vi "toString.vi"(10 "Variant":variant, 11 "StringFormatter in":refnum<class "StringFormatter.lvclass">) -> (0 "error out":errorcluster, 2 "Value":string)   [LabVIEW 2013, in "OpenStringFormatter.lvlib" / "StringFormatter.lvclass"]
uses:
  StringFormatter.lvclass
  StringFormatter.lvclass/StringFormatter.ctl
  TypeDescriptor/OpenDescriptor.lvlib
  Conversions/OpenConvert.lvlib
  Variant/OpenVariant.lvlib
panel:
  out "interleaved array (noUnits)":u8[](array[numeric]) format="%.0x"
  out "x = y?":bool
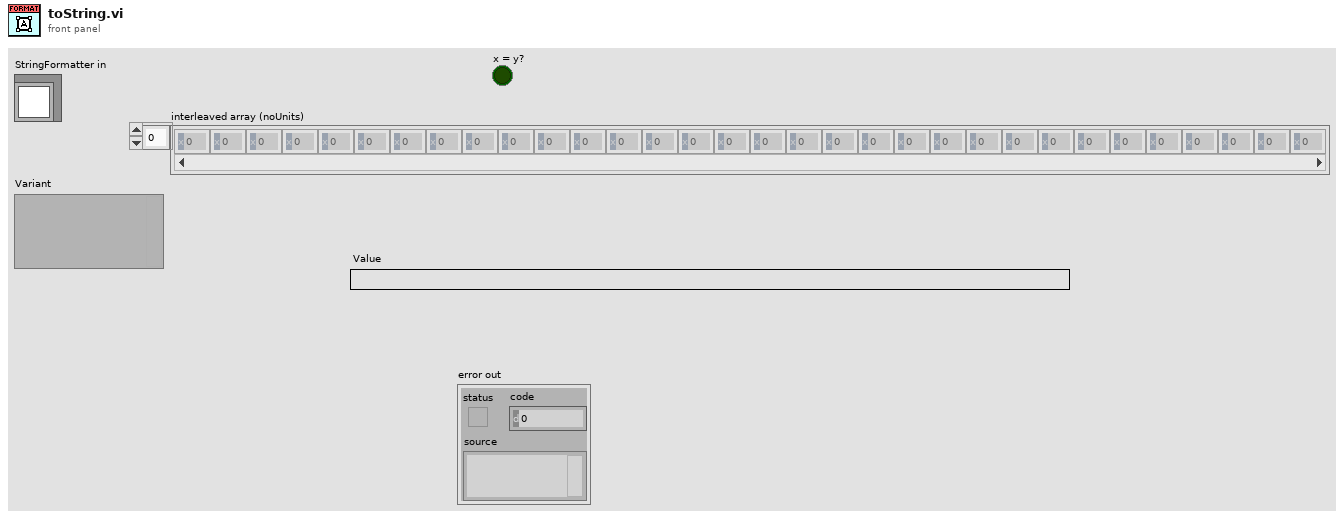
[diagram p1: front panel]
types:
  T1 = typedef "OpenStringFormatter.lvlib/StringFormatter.lvclass/Localization Decimal Separator -- enum.ctl" = enum16{"System", "Comma", "Dot"}
  T2 = typedef "VariantType.lvlib/UnitInfo.ctl" = cluster{"UnitType":T3, "Exponent":i16}
  T3 = typedef "VariantType.lvlib/UnitType.ctl" = enum16{"Radians", "Steradians", "Seconds", "Meters", "Kilograms", "Amperes", "Kelvins", "Moles", "Candelas", "InvalidUnit"}
  T4 = typedef "Type Enum.ctl" = enum8{"Void", "I8", "I16", "I32", "I64", "U8", "U16", "U32", "U64", "Single Float", "Double Float", "Extended Float", "Single Complex", "Double Complex", "Extended Complex", "Enum I8 NEVER", "Enum I16 NEVER", "Enum I32 NEVER", "Enum I64 NEVER", "Enum U8", "Enum U16", "Enum U32", "Enum U64", "Single Float With Unit", "Double Float With Unit", "Extended Float With Unit", "Single Complex With Unit", "Double Complex With Unit", "Extended Complex With Unit", "boolU16", "Boolean", "String", "Handle", "Path", "Picture", "C String", "Pascal String", "Tag", "SubString", "Array", "SubArray", "Cluster", "Numeric Cluster", "Variant", "LV Variant", "Measure Data (waveform)", "Refnum", "ExtData", "function", "Typedef", "Poly VI", "bad wire", "LabVIEW Class Instance"}
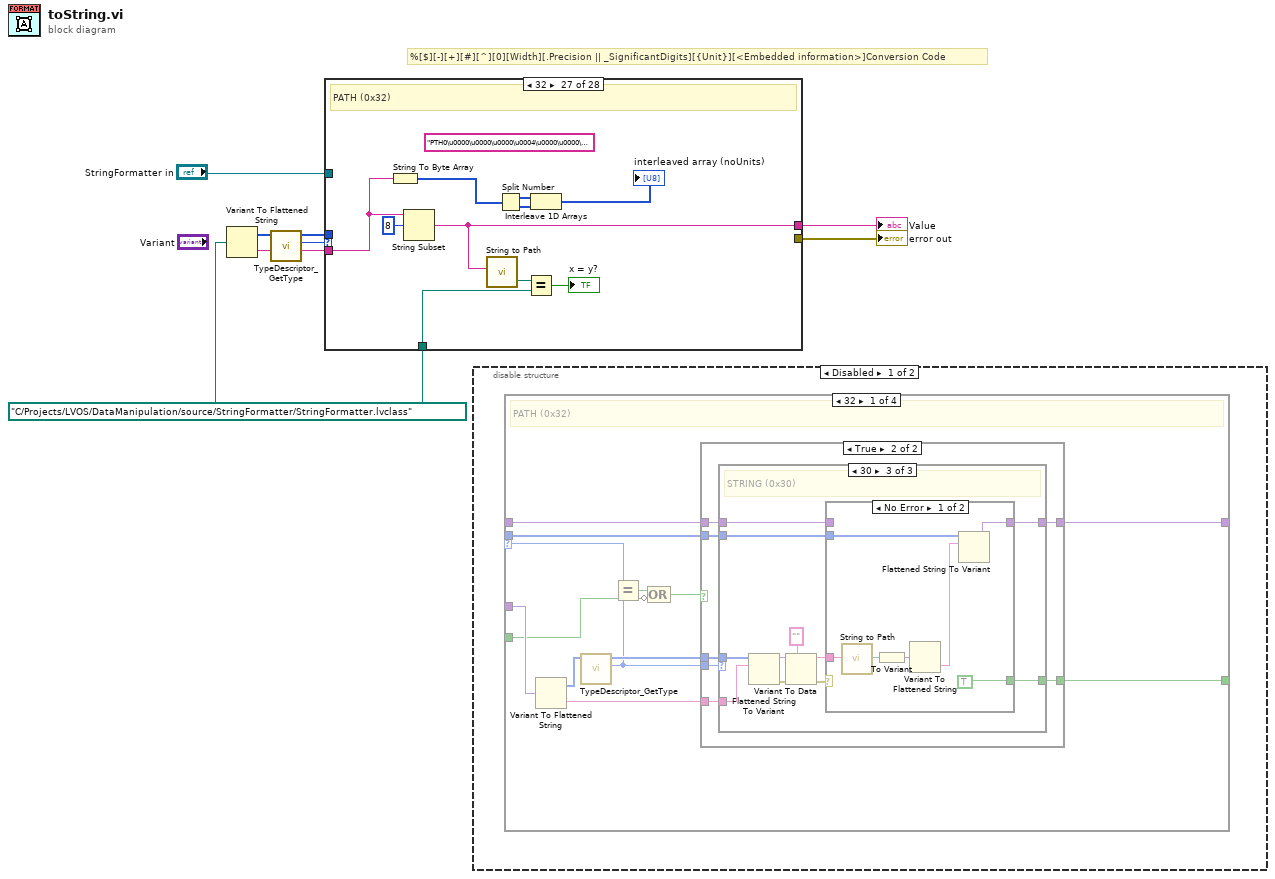
[diagram p0: block diagram]
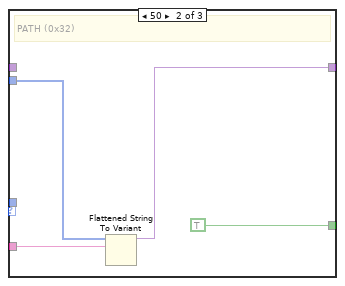
[diagram p4: hidden frame]
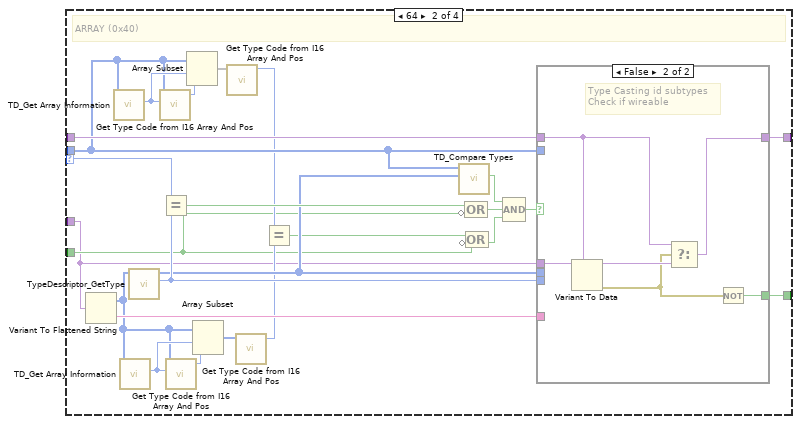
[diagram p6: hidden frame]
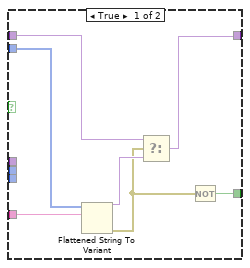
[diagram p7: hidden frame]
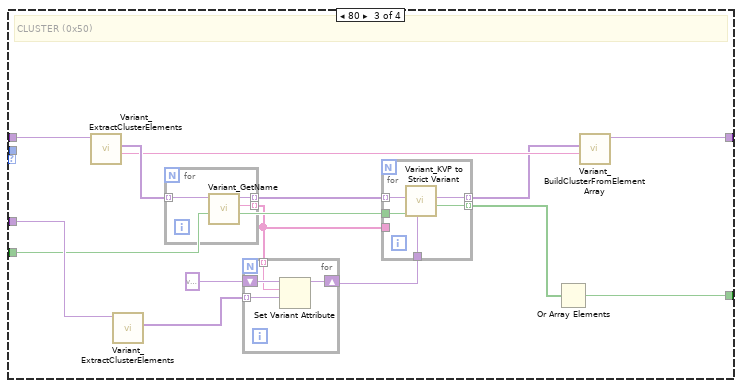
[diagram p8: hidden frame]
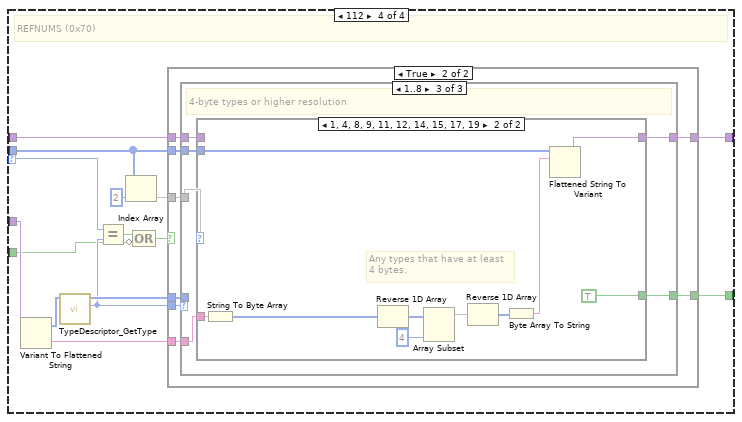
[diagram p9: hidden frame]
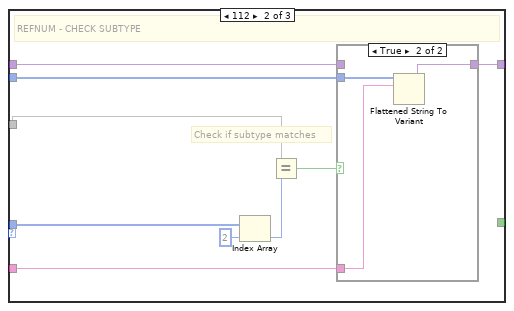
[diagram p12: hidden frame]
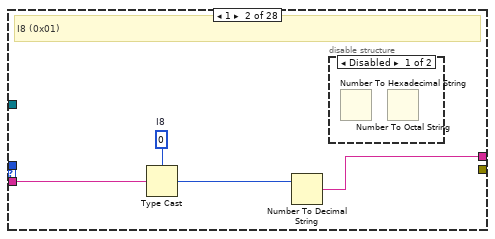
[diagram p17: hidden frame]
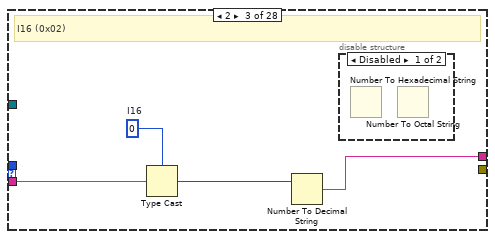
[diagram p19: hidden frame]
diagram:
  w1 = path "C:/Projects/LVOS/DataManipulation/source/StringFormatter/StringFormatter.lvclass"
  # "%[$][-][+][#][^][0][Width][.Precision || _SignificantDigits][{Unit}][<Embedded information>]Conversion Code"
  n1 = Variant To Flattened String(Variant=w1) -> (data string=w3:string, 1:w5:i16[])
  n2 = call "TypeDescriptor_GetType.vi"("type descriptor"=w5) -> ("Type"=w4:u8, "type descriptor dup"=w2:i16[])  [unwired: 9 in]
  n3 = case shown="32" w4 {
    tunnel: [_ w11 w15 w19 w23 w27 w31 w35 w39 w42 w52 w62 w76 w87 w97 w105 w119 w133 w147 w163 w178 w193 w208 w223 w233 w239 w250 w254] -> w8
    tunnel: [_ _ _ _ _ _ _ _ _ _ _ _ _ _ _ _ _ _ _ _ _ _ _ _ _ _ _ w253] -> w7
    tunnel: w3 -> [_ w10 w13 w17 w21 w25 w29 w33 w37 w48 w59 w69 w79 w89 w99 w107 w121 w135 w157 w172 w187 w202 w217 w232 w238 w240 w246 w252]
    tunnel: "StringFormatter in" -> [_ _ _ _ _ _ _ _ _ w49 w60 w70 w80 w90 w100 w103 w117 w130 w152 w168 w183 w198 w213 w228 _ _ _ _]
    tunnel: w2 -> [_ _ _ _ _ _ _ _ _ _ _ _ _ _ _ w104 w118 w131 w150 w166 w181 w196 w211 w226 _ _ _ _]
    tunnel: w1 -> [_ _ _ _ _ _ _ _ _ _ _ _ _ _ _ _ _ _ _ _ _ _ _ _ _ _ w248 _]
    frame 0 {
    }
    frame 1 {
      w9 = i8 0  # I8
      # "I8 (0x01)"
      n4 = Type Cast(type=w9, x=w10) -> (*(type *) &x=w12:i8)
      n5 = Number To Decimal String(number=w12) -> (decimal integer string=w11:string)  [unwired: 1 in]
      n6 = disable-structure shown="Disabled" {
        frame Disabled {
          n7 = Number To Hexadecimal String() -> ()  [unwired: 2 in, 1 out]
          n8 = Number To Octal String() -> ()  [unwired: 2 in, 1 out]
        }
        frame Enabled {
        }
      }
    }
    frame 2 {
      w14 = i16 0  # I16
      # "I16 (0x02)"
      n9 = Type Cast(type=w14, x=w13) -> (*(type *) &x=w16:i16)
      n10 = Number To Decimal String(number=w16) -> (decimal integer string=w15:string)  [unwired: 1 in]
      n11 = disable-structure shown="Disabled" {
        frame Disabled {
          n12 = Number To Hexadecimal String() -> ()  [unwired: 2 in, 1 out]
          n13 = Number To Octal String() -> ()  [unwired: 2 in, 1 out]
        }
        frame Enabled {
        }
      }
    }
    frame 3 {
      w18 = 0  # I32
      # "I32 (0x03)"
      n14 = Type Cast(type=w18, x=w17) -> (*(type *) &x=w20:i32)
      n15 = Number To Decimal String(number=w20) -> (decimal integer string=w19:string)  [unwired: 1 in]
      n16 = disable-structure shown="Disabled" {
        frame Disabled {
          n17 = Number To Hexadecimal String() -> ()  [unwired: 2 in, 1 out]
          n18 = Number To Octal String() -> ()  [unwired: 2 in, 1 out]
        }
        frame Enabled {
        }
      }
    }
    frame 4 {
      w22 = i64 0  # I64
      # "I64 (0x04)"
      n19 = Type Cast(type=w22, x=w21) -> (*(type *) &x=w24:i64)
      n20 = Number To Decimal String(number=w24) -> (decimal integer string=w23:string)  [unwired: 1 in]
      n21 = disable-structure shown="Disabled" {
        frame Disabled {
          n22 = Number To Hexadecimal String() -> ()  [unwired: 2 in, 1 out]
          n23 = Number To Octal String() -> ()  [unwired: 2 in, 1 out]
        }
        frame Enabled {
        }
      }
    }
    frame 5 {
      w26 = u8 0  # U8
      # "U8 (0x05)"
      n24 = Type Cast(type=w26, x=w25) -> (*(type *) &x=w28:u8)
      n25 = Number To Decimal String(number=w28) -> (decimal integer string=w27:string)  [unwired: 1 in]
      n26 = disable-structure shown="Disabled" {
        frame Disabled {
          n27 = Number To Hexadecimal String() -> ()  [unwired: 2 in, 1 out]
          n28 = Number To Octal String() -> ()  [unwired: 2 in, 1 out]
        }
        frame Enabled {
        }
      }
    }
    frame 6 {
      w30 = u16 0  # U16
      # "U16 (0x06)"
      n29 = Type Cast(type=w30, x=w29) -> (*(type *) &x=w32:u16)
      n30 = Number To Decimal String(number=w32) -> (decimal integer string=w31:string)  [unwired: 1 in]
      n31 = disable-structure shown="Disabled" {
        frame Disabled {
          n32 = Number To Hexadecimal String() -> ()  [unwired: 2 in, 1 out]
          n33 = Number To Octal String() -> ()  [unwired: 2 in, 1 out]
        }
        frame Enabled {
        }
      }
    }
    frame 7 {
      w34 = u32 0  # U32
      # "U32 (0x07)"
      n34 = Type Cast(type=w34, x=w33) -> (*(type *) &x=w36:u32)
      n35 = Number To Decimal String(number=w36) -> (decimal integer string=w35:string)  [unwired: 1 in]
      n36 = disable-structure shown="Disabled" {
        frame Disabled {
          n37 = Number To Hexadecimal String() -> ()  [unwired: 2 in, 1 out]
          n38 = Number To Octal String() -> ()  [unwired: 2 in, 1 out]
        }
        frame Enabled {
        }
      }
    }
    frame 8 {
      w38 = u64 0  # U64
      # "U64 (0x08)"
      n39 = Type Cast(type=w38, x=w37) -> (*(type *) &x=w40:u64)
      n40 = Number To Decimal String(number=w40) -> (decimal integer string=w39:string)  [unwired: 1 in]
      n41 = disable-structure shown="Disabled" {
        frame Disabled {
          n42 = Number To Hexadecimal String() -> ()  [unwired: 2 in, 1 out]
          n43 = Number To Octal String() -> ()  [unwired: 2 in, 1 out]
        }
        frame Enabled {
        }
      }
    }
    frame 9 {
      w50 = sgl 0.0  # SGL
      # "SGL (0x09)"
      n44 = call "Read Decimal Separator.vi"("StringFormatter in"=w49) -> ("Decimal Separator"=w44:T1, "StringFormatter out"=w41:refnum<class "StringFormatter.lvclass">)  [unwired: 9 in]
      n45 = call-dynamic "getDecimalSeparatorString.vi"("Decimal Separator"=w44, "StringFormatter"=w41) -> ("Formatter String"=w47:string)  [unwired: 9 in]
      n46 = Type Cast(type=w50, x=w48) -> (*(type *) &x=w43:sgl)
      n47 = Concatenate Strings(w47, "%#g" ("string")) -> (w46:string)
      n48 = Format Value(format string=w46, value (0)=w43) -> (output string=w42:string)  [unwired: 1 in]
    }
    frame 10 {
      w58 = 0.0  # DBL
      # "DBL (0xA)"
      n49 = call "Read Decimal Separator.vi"("StringFormatter in"=w60) -> ("Decimal Separator"=w54:T1, "StringFormatter out"=w51:refnum<class "StringFormatter.lvclass">)  [unwired: 9 in]
      n50 = call-dynamic "getDecimalSeparatorString.vi"("Decimal Separator"=w54, "StringFormatter"=w51) -> ("Formatter String"=w57:string)  [unwired: 9 in]
      n51 = Type Cast(type=w58, x=w59) -> (*(type *) &x=w53:dbl)
      n52 = Concatenate Strings(w57, "%#g" ("string")) -> (w56:string)
      n53 = Format Value(format string=w56, value (0)=w53) -> (output string=w52:string)  [unwired: 1 in]
    }
    frame 11 {
      w68 = ext 0.0  # EXT
      # "EXT (0x0B)"
      n54 = call "Read Decimal Separator.vi"("StringFormatter in"=w70) -> ("Decimal Separator"=w64:T1, "StringFormatter out"=w61:refnum<class "StringFormatter.lvclass">)  [unwired: 9 in]
      n55 = call-dynamic "getDecimalSeparatorString.vi"("Decimal Separator"=w64, "StringFormatter"=w61) -> ("Formatter String"=w67:string)  [unwired: 9 in]
      n56 = Type Cast(type=w68, x=w69) -> (*(type *) &x=w63:ext)
      n57 = Concatenate Strings(w67, "%#g" ("string")) -> (w66:string)
      n58 = Format Value(format string=w66, value (0)=w63) -> (output string=w62:string)  [unwired: 1 in]
    }
    frame 12 {
      w78 = csg 0.0+0.0i  # CSG
      # "CSG (0x0C)"
      n59 = call "Read Decimal Separator.vi"("StringFormatter in"=w80) -> ("Decimal Separator"=w75:T1, "StringFormatter out"=w71:refnum<class "StringFormatter.lvclass">)  [unwired: 9 in]
      n60 = Type Cast(type=w78, x=w79) -> (*(type *) &x=w77:csg)
      n61 = call-dynamic "getDecimalSeparatorString.vi"("Decimal Separator"=w75, "StringFormatter"=w71) -> ("Formatter String"=w74:string)  [unwired: 9 in]
      n62 = Concatenate Strings(w74, "%#g" ("string")) -> (w73:string)
      n63 = Format Value(format string=w73, value (0)=w77) -> (output string=w76:string)  [unwired: 1 in]
    }
    frame 13 {
      w82 = cdb 0.0+0.0i  # CDB
      # "CDB (0x0D)"
      n64 = call "Read Decimal Separator.vi"("StringFormatter in"=w90) -> ("Decimal Separator"=w86:T1, "StringFormatter out"=w81:refnum<class "StringFormatter.lvclass">)  [unwired: 9 in]
      n65 = Type Cast(type=w82, x=w89) -> (*(type *) &x=w88:cdb)
      n66 = call-dynamic "getDecimalSeparatorString.vi"("Decimal Separator"=w86, "StringFormatter"=w81) -> ("Formatter String"=w85:string)  [unwired: 9 in]
      n67 = Concatenate Strings(w85, "%#g" ("string")) -> (w84:string)
      n68 = Format Value(format string=w84, value (0)=w88) -> (output string=w87:string)  [unwired: 1 in]
    }
    frame 14 {
      w92 = cxt 0.0+0.0i  # CXT
      # "CXT (0x0E)"
      n69 = call "Read Decimal Separator.vi"("StringFormatter in"=w100) -> ("Decimal Separator"=w96:T1, "StringFormatter out"=w91:refnum<class "StringFormatter.lvclass">)  [unwired: 9 in]
      n70 = Type Cast(type=w92, x=w99) -> (*(type *) &x=w98:cxt)
      n71 = call-dynamic "getDecimalSeparatorString.vi"("Decimal Separator"=w96, "StringFormatter"=w91) -> ("Formatter String"=w95:string)  [unwired: 9 in]
      n72 = Concatenate Strings(w95, "%#g" ("string")) -> (w94:string)
      n73 = Format Value(format string=w94, value (0)=w98) -> (output string=w97:string)  [unwired: 1 in]
    }
    frame 21 {
      w101 = u8 0  # U8
      # "Enum U8 (0x15)"
      n74 = call "Read enum as string.vi"("StringFormatter in"=w103) -> ("enum as string"=w102:bool)  [unwired: 9 in, 1 out]
      n75 = Type Cast(type=w101, x=w107) -> (*(type *) &x=w106:u8)
      n76 = case shown="True" w102 {
        tunnel: w106 -> [w110 w112]
        tunnel: [w109 w111] -> w105
        tunnel: w104 -> [_ w114]
        frame False {
          n77 = Format Value(format string="%d", value (0)=w110) -> (output string=w109:string)  [unwired: 1 in]
        }
        frame True {
          n78 = call "TypeDescriptor_ListElementNames.vi"("type descriptor"=w114) -> ("element names"=w113:string[])  [unwired: 7 in, 3 out]
          n79 = Index Array(array=w113, index=w112) -> (element=w111:string)
        }
      }
    }
    frame 22 {
      w115 = u16 0  # U16
      # "Enum U16 (0x16)"
      n80 = call "Read enum as string.vi"("StringFormatter in"=w117) -> ("enum as string"=w116:bool)  [unwired: 9 in, 1 out]
      n81 = Type Cast(type=w115, x=w121) -> (*(type *) &x=w120:u16)
      n82 = case shown="True" w116 {
        tunnel: w120 -> [w124 w126]
        tunnel: [w123 w125] -> w119
        tunnel: w118 -> [_ w128]
        frame False {
          n83 = Format Value(format string="%d", value (0)=w124) -> (output string=w123:string)  [unwired: 1 in]
        }
        frame True {
          n84 = call "TypeDescriptor_ListElementNames.vi"("type descriptor"=w128) -> ("element names"=w127:string[])  [unwired: 7 in, 3 out]
          n85 = Index Array(array=w127, index=w126) -> (element=w125:string)
        }
      }
    }
    frame 23 {
      w132 = u32 0  # U32
      # "Enum U32 (0x17)"
      n86 = call "Read enum as string.vi"("StringFormatter in"=w130) -> ("enum as string"=w129:bool)  [unwired: 9 in, 1 out]
      n87 = Type Cast(type=w132, x=w135) -> (*(type *) &x=w134:u32)
      n88 = case shown="True" w129 {
        tunnel: w134 -> [w138 w140]
        tunnel: [w137 w139] -> w133
        tunnel: w131 -> [_ w142]
        frame False {
          n89 = Format Value(format string="%d", value (0)=w138) -> (output string=w137:string)  [unwired: 1 in]
        }
        frame True {
          n90 = call "TypeDescriptor_ListElementNames.vi"("type descriptor"=w142) -> ("element names"=w141:string[])  [unwired: 7 in, 3 out]
          n91 = Index Array(array=w141, index=w140) -> (element=w139:string)
        }
      }
    }
    frame 25 {
      w155 = sgl 0.0  # SGL
      # "SGL PhysUnit (0x19)"
      n92 = call "Read Decimal Separator.vi"("StringFormatter in"=w152) -> ("Decimal Separator"=w151:T1, "StringFormatter out"=w143:refnum<class "StringFormatter.lvclass">)  [unwired: 9 in]
      n93 = call "TypeDescriptor_GetUnits.vi"("type descriptor"=w150) -> ("Units"=w145:T2[])  [unwired: 8 in, 2 out]
      n94 = Type Cast(type=w155, x=w157) -> (*(type *) &x=w156:sgl)
      n95 = call-dynamic "formatUnits.vi"("Units"=w145, "StringFormatter"=w143) -> ("Units String"=w144:string)  [unwired: 9 in]
      n96 = call-dynamic "getDecimalSeparatorString.vi"("Decimal Separator"=w151, "StringFormatter"=w143) -> ("Formatter String"=w154:string)  [unwired: 9 in]
      n97 = Concatenate Strings(w154, "%#g" ("string")) -> (w149:string)
      n98 = Format Value(format string=w149, value (0)=w156) -> (output string=w148:string)  [unwired: 1 in]
      n99 = call <vilib>:"Space Constant.vi"() -> ("String"=w146:string)
      n100 = Concatenate Strings(w148, w146, w144) -> (w147:string)
    }
    frame 26 {
      w158 = 0.0  # DBL
      # "DBL PhysUnit (0x1A)"
      n101 = call "Read Decimal Separator.vi"("StringFormatter in"=w168) -> ("Decimal Separator"=w167:T1, "StringFormatter out"=w159:refnum<class "StringFormatter.lvclass">)  [unwired: 9 in]
      n102 = call "TypeDescriptor_GetUnits.vi"("type descriptor"=w166) -> ("Units"=w161:T2[])  [unwired: 8 in, 2 out]
      n103 = Type Cast(type=w158, x=w172) -> (*(type *) &x=w171:dbl)
      n104 = call-dynamic "formatUnits.vi"("Units"=w161, "StringFormatter"=w159) -> ("Units String"=w160:string)  [unwired: 9 in]
      n105 = call-dynamic "getDecimalSeparatorString.vi"("Decimal Separator"=w167, "StringFormatter"=w159) -> ("Formatter String"=w170:string)  [unwired: 9 in]
      n106 = Concatenate Strings(w170, "%#g" ("string")) -> (w165:string)
      n107 = Format Value(format string=w165, value (0)=w171) -> (output string=w164:string)  [unwired: 1 in]
      n108 = call <vilib>:"Space Constant.vi"() -> ("String"=w162:string)
      n109 = Concatenate Strings(w164, w162, w160) -> (w163:string)
    }
    frame 27 {
      w173 = ext 0.0  # EXT
      # "EXT PhysUnit (0x1B)"
      n110 = call "Read Decimal Separator.vi"("StringFormatter in"=w183) -> ("Decimal Separator"=w182:T1, "StringFormatter out"=w174:refnum<class "StringFormatter.lvclass">)  [unwired: 9 in]
      n111 = call "TypeDescriptor_GetUnits.vi"("type descriptor"=w181) -> ("Units"=w176:T2[])  [unwired: 8 in, 2 out]
      n112 = Type Cast(type=w173, x=w187) -> (*(type *) &x=w186:ext)
      n113 = call-dynamic "formatUnits.vi"("Units"=w176, "StringFormatter"=w174) -> ("Units String"=w175:string)  [unwired: 9 in]
      n114 = call-dynamic "getDecimalSeparatorString.vi"("Decimal Separator"=w182, "StringFormatter"=w174) -> ("Formatter String"=w185:string)  [unwired: 9 in]
      n115 = Concatenate Strings(w185, "%#g" ("string")) -> (w180:string)
      n116 = Format Value(format string=w180, value (0)=w186) -> (output string=w179:string)  [unwired: 1 in]
      n117 = call <vilib>:"Space Constant.vi"() -> ("String"=w177:string)
      n118 = Concatenate Strings(w179, w177, w175) -> (w178:string)
    }
    frame 28 {
      w188 = csg 0.0+0.0i  # CSG
      # "CSG PhysUnit (0x1C)"
      n119 = call "Read Decimal Separator.vi"("StringFormatter in"=w198) -> ("Decimal Separator"=w197:T1, "StringFormatter out"=w189:refnum<class "StringFormatter.lvclass">)  [unwired: 9 in]
      n120 = call "TypeDescriptor_GetUnits.vi"("type descriptor"=w196) -> ("Units"=w191:T2[])  [unwired: 8 in, 2 out]
      n121 = Type Cast(type=w188, x=w202) -> (*(type *) &x=w201:csg)
      n122 = call-dynamic "formatUnits.vi"("Units"=w191, "StringFormatter"=w189) -> ("Units String"=w190:string)  [unwired: 9 in]
      n123 = call-dynamic "getDecimalSeparatorString.vi"("Decimal Separator"=w197, "StringFormatter"=w189) -> ("Formatter String"=w200:string)  [unwired: 9 in]
      n124 = Concatenate Strings(w200, "%#g" ("string")) -> (w195:string)
      n125 = Format Value(format string=w195, value (0)=w201) -> (output string=w194:string)  [unwired: 1 in]
      n126 = call <vilib>:"Space Constant.vi"() -> ("String"=w192:string)
      n127 = Concatenate Strings(w194, w192, w190) -> (w193:string)
    }
    frame 29 {
      w203 = cdb 0.0+0.0i  # CDB
      # "CDB PhysUnit (0x1D)"
      n128 = call "Read Decimal Separator.vi"("StringFormatter in"=w213) -> ("Decimal Separator"=w212:T1, "StringFormatter out"=w204:refnum<class "StringFormatter.lvclass">)  [unwired: 9 in]
      n129 = call "TypeDescriptor_GetUnits.vi"("type descriptor"=w211) -> ("Units"=w206:T2[])  [unwired: 8 in, 2 out]
      n130 = Type Cast(type=w203, x=w217) -> (*(type *) &x=w216:cdb)
      n131 = call-dynamic "formatUnits.vi"("Units"=w206, "StringFormatter"=w204) -> ("Units String"=w205:string)  [unwired: 9 in]
      n132 = call-dynamic "getDecimalSeparatorString.vi"("Decimal Separator"=w212, "StringFormatter"=w204) -> ("Formatter String"=w215:string)  [unwired: 9 in]
      n133 = Concatenate Strings(w215, "%#g" ("string")) -> (w210:string)
      n134 = Format Value(format string=w210, value (0)=w216) -> (output string=w209:string)  [unwired: 1 in]
      n135 = call <vilib>:"Space Constant.vi"() -> ("String"=w207:string)
      n136 = Concatenate Strings(w209, w207, w205) -> (w208:string)
    }
    frame 30 {
      w218 = cxt 0.0+0.0i  # CXT
      # "CXT PhysUnit (0x1E)"
      n137 = call "Read Decimal Separator.vi"("StringFormatter in"=w228) -> ("Decimal Separator"=w227:T1, "StringFormatter out"=w219:refnum<class "StringFormatter.lvclass">)  [unwired: 9 in]
      n138 = call "TypeDescriptor_GetUnits.vi"("type descriptor"=w226) -> ("Units"=w221:T2[])  [unwired: 8 in, 2 out]
      n139 = Type Cast(type=w218, x=w232) -> (*(type *) &x=w231:cxt)
      n140 = call-dynamic "formatUnits.vi"("Units"=w221, "StringFormatter"=w219) -> ("Units String"=w220:string)  [unwired: 9 in]
      n141 = call-dynamic "getDecimalSeparatorString.vi"("Decimal Separator"=w227, "StringFormatter"=w219) -> ("Formatter String"=w230:string)  [unwired: 9 in]
      n142 = Concatenate Strings(w230, "%#g" ("string")) -> (w225:string)
      n143 = Format Value(format string=w225, value (0)=w231) -> (output string=w224:string)  [unwired: 1 in]
      n144 = call <vilib>:"Space Constant.vi"() -> ("String"=w222:string)
      n145 = Concatenate Strings(w224, w222, w220) -> (w223:string)
    }
    frame 33 {
      # "Boolean (0x21)"
      n146 = Type Cast(type=FALSE, x=w238) -> (*(type *) &x=w236:bool)
      n147 = Select(t="true", s=w236, f="false") -> (s? t:f=w233:string)
    }
    frame 48 {
      # "STRING (0x30)"
      n148 = String Subset(string=w240, offset (0)=4) -> (substring=w239:string)  [unwired: 1 in]
    }
    frame 50 {
      (unwired) "PTH0\u0000\u0000\u0000\u0004\u0000\u0000\u0000\u0000" ("string")
      # "PATH (0x32)"
      n149 = String To Byte Array(string=w246) -> (unsigned byte array=w243:u8[])
      n150 = String Subset(string=w246, offset (0)=8) -> (substring=w250:string)  [unwired: 1 in]
      n151 = call "String to Path.vi"("common path"=w250) -> ("specific path"=w249:path)  [unwired: 10 in]
      n152 = Split Number(x=w243) -> (hi(x)=w244:u8[], lo(x)=w245:u8[])
      n153 = Equal?(x=w249, y=w248) -> (x = y?=→"x = y?":bool)
      n154 = Interleave 1D Arrays(w244, w245) -> (→"interleaved array (noUnits)":u8[])
    }
    frame Default {
      n155 = call <userlib>:"Format Variant Into String__ogtk.vi"("Variant"=w252) -> ("Output String"=w254:string, "error out"=w253:errorcluster)  [unwired: 13 in]
    }
  }
  "error out" <- w7
  "Value" <- w8
  n156 = disable-structure shown="Disabled" {
    frame Disabled {
      n157 = case shown="32" {
        selector: _ -> [w258 w319 _ w364]
        tunnel: _ -> [w267 w300 w350 w378]
        tunnel: [w263 w322 w342 w374] -> _
        tunnel: _ -> [w264 w323 w351 w375]
        tunnel: _ -> [w262 w314 _ w371]
        tunnel: [w260 w321 w343 w369] -> _
        tunnel: _ -> [w256 w302 w347 w366]
        frame 50 {
          # "PATH (0x32)"
          n158 = Variant To Flattened String(Variant=w267) -> (data string=w266:string, 1:w265:i16[])
          n159 = call "TypeDescriptor_GetType.vi"("type descriptor"=w265) -> ("Type"=w257:u8, "type descriptor dup"=w261:i16[])  [unwired: 9 in]
          n160 = Equal?(x=w258, y=w257) -> (x = y?=w259:bool)
          n161 = Compound Arithmetic op=OR(w259, invert w256) -> (w255:bool)
          n162 = case shown="True" w255 {
            tunnel: w266 -> [_ w275]
            tunnel: w264 -> [w268 w274]
            tunnel: [w268 w273] -> w263
            tunnel: w262 -> [_ w272]
            tunnel: w261 -> [_ w271]
            tunnel: [_ w270] -> w260
            tunnel: w257 -> [_ w269]
            frame False {
            }
            frame True {
              n163 = case shown="30" w269 {
                tunnel: w275 -> [_ w280 w289]
                tunnel: w274 -> [w276 _ w283]
                tunnel: [w276 w279 w285] -> w273
                tunnel: w272 -> [_ w278 w291]
                tunnel: w271 -> [_ _ w290]
                tunnel: [_ TRUE w281] -> w270
                frame Default {
                  # "INCOMPATIBLE DATATYPES"
                }
                frame 50 {
                  # "PATH (0x32)"
                  n164 = Flattened String To Variant(6:w280, 7:w278) -> (3:w279:variant)  [unwired: 1 in, 1 out]
                }
                frame 48 {
                  # "STRING (0x30)"
                  n165 = Flattened String To Variant(6:w289, 7:w290) -> (0:w286:errorcluster, 3:w288:variant)  [unwired: 1 in]
                  n166 = Variant To Data(error in=w286, type="", Variant=w288) -> (data=w282:string, error out=w284:errorcluster)
                  n167 = case shown="No Error" w284 {
                    tunnel: w291 -> [w298 _]
                    tunnel: [w297 w299] -> w285
                    tunnel: w283 -> [_ w299]
                    tunnel: w282 -> [w293 _]
                    tunnel: [TRUE _] -> w281
                    frame No Error {
                      n168 = call "String to Path.vi"("common path"=w293) -> ("specific path"=w292:path)  [unwired: 10 in]
                      n169 = To Variant(anything=w292) -> (Variant=w296:variant)
                      n170 = Variant To Flattened String(Variant=w296) -> (data string=w295:string)  [unwired: 1 out]
                      n171 = Flattened String To Variant(6:w295, 7:w298) -> (3:w297:variant)  [unwired: 1 in, 1 out]
                    }
                    frame Error {
                    }
                  }
                }
              }
            }
          }
        }
        frame 64 {
          # "ARRAY (0x40)"
          n172 = Variant To Flattened String(Variant=w300) -> (data string=w324:string, 1:w307:i16[])
          n173 = call <vilib>:"TD_Get Array Information.vi"("Type descriptor"=w314) -> ("Contained TD Offset"=w317:i32)  [unwired: 8 in, 2 out]
          n174 = call <vilib>:"TD_Get Array Information.vi"("Type descriptor"=w307) -> ("Contained TD Offset"=w308:i32)  [unwired: 8 in, 2 out]
          n175 = call "TypeDescriptor_GetType.vi"("type descriptor"=w307) -> ("Type"=w318:u8, "type descriptor dup"=w313:i16[])  [unwired: 9 in]
          n176 = call <vilib>:"Get Type Code from I16 Array And Pos.vi"("Pos in Type Descriptor (0)"=w317, "Type descriptor"=w314) -> ("Size (Words)"=w316:i32)  [unwired: 7 in, 2 out]
          n177 = Equal?(x=w319, y=w318) -> (x = y?=w320:bool)
          n178 = call <vilib>:"Get Type Code from I16 Array And Pos.vi"("Pos in Type Descriptor (0)"=w308, "Type descriptor"=w307) -> ("Size (Words)"=w309:i32)  [unwired: 7 in, 2 out]
          n179 = Array Subset(array=w314, index=w317, length=w316) -> (w315:void[])
          n180 = Array Subset(array=w307, index=w308, length=w309) -> (w310:i16[])
          n181 = call <vilib>:"Get Type Code from I16 Array And Pos.vi"("Type descriptor"=w315) -> ("Type Enum"=w306:T4)  [unwired: 8 in, 2 out]
          n182 = call <vilib>:"Get Type Code from I16 Array And Pos.vi"("Type descriptor"=w310) -> ("Type Enum"=w305:T4)  [unwired: 8 in, 2 out]
          n183 = Equal?(x=w306, y=w305) -> (x = y?=w303:bool)
          n184 = call <vilib>:"TD_Compare Types.vi"("Type descriptor 2"=w313, "Type descriptor"=w314) -> ("Types Wireable?"=w312:bool)  [unwired: 9 in]
          n185 = Compound Arithmetic op=OR(w320, invert w302) -> (w304:bool)
          n186 = Compound Arithmetic op=OR(w303, invert w302) -> (w301:bool)
          n187 = Compound Arithmetic op=AND(w312, w304, w301) -> (w311:bool)
          n188 = case shown="False" w311 {
            tunnel: w324 -> [w331 _]
            tunnel: w323 -> [w329 w334]
            tunnel: [w327 w337] -> w322
            tunnel: w314 -> [w330 _]
            tunnel: w313 -> [_ _]
            tunnel: [w325 w336] -> w321
            tunnel: w318 -> [_ _]
            tunnel: w300 -> [_ w335]
            frame True {
              n189 = Flattened String To Variant(6:w331, 7:w330) -> (0:w326:errorcluster, 3:w328:variant)  [unwired: 1 in]
              n190 = Select(t=w329, s=w326, f=w328) -> (s? t:f=w327:variant)
              n191 = Not(x=w326) -> (.not. x?=w325:bool)
            }
            frame False {
              # "Type Casting id subtypes\nCheck if wireable"
              n192 = Variant To Data(type=w334, Variant=w335) -> (data=w333:variant, error out=w332:errorcluster)  [unwired: 1 in]
              n193 = Select(t=w334, s=w332, f=w333) -> (s? t:f=w337:variant)
              n194 = Not(x=w332) -> (.not. x?=w336:bool)
            }
          }
        }
        frame 80 {
          # "CLUSTER (0x50)"
          n195 = call "Variant_ExtractClusterElements.vi"("Cluster"=w351) -> ("name"=w348:string, "Elements"=w349:variant[])  [unwired: 8 in, 1 out]
          n196 = call "Variant_ExtractClusterElements.vi"("Cluster"=w350) -> ("Elements"=w339:variant[])  [unwired: 8 in, 2 out]
          n197 = for {
            tunnel: w349 -> [w363] mode=indexing
            tunnel: [w362] -> w340 mode=indexing
            tunnel: [w361] -> w346 mode=indexing
            n198 = call "Variant_GetName.vi"("Variant"=w363) -> ("Name"=w362:string, "Variant dup"=w361:variant)  [unwired: 8 in, 1 out]
          }
          n199 = for {
            shift-right: [w354] -> w338
            shift-left: variant ("variant") -> [w355]
            tunnel: w340 -> [w353] mode=indexing
            tunnel: w339 -> [w352] mode=indexing
            n200 = Set Variant Attribute(Variant=w355, name=w353, value=w352) -> (Variant out=w354:variant)  [unwired: 1 in, 2 out]
          }
          n201 = for {
            tunnel: w347 -> [w360]
            tunnel: w346 -> [w359] mode=indexing
            tunnel: [w358] -> w345 mode=indexing
            tunnel: [w357] -> w344 mode=indexing
            tunnel: w340 -> [_]
            tunnel: w338 -> [w356]
            n202 = call "Variant_KVP to Strict Variant.vi"("KVP"=w356, "Strict type matching? (F)"=w360, "Default Value"=w359) -> ("any found?"=w357:bool, "Value"=w358:variant)  [unwired: 5 in, 2 out]
          }
          n203 = Or Array Elements(Boolean array=w344) -> (logical OR=w343:bool)
          n204 = call "Variant_BuildClusterFromElementArray.vi"("name"=w348, "Elements"=w345) -> ("Cluster"=w342:variant)  [unwired: 9 in]
        }
        frame 112 {
          # "REFNUMS (0x70)"
          n205 = Variant To Flattened String(Variant=w378) -> (data string=w377:string, 1:w376:i16[])
          n206 = call "TypeDescriptor_GetType.vi"("type descriptor"=w376) -> ("Type"=w368:u8, "type descriptor dup"=w373:i16[])  [unwired: 9 in]
          n207 = Equal?(x=w364, y=w368) -> (x = y?=w367:bool)
          n208 = Index Array(array=w371, index=2) -> (element=w370)
          n209 = Compound Arithmetic op=OR(w367, invert w366) -> (w365:bool)
          n210 = case shown="True" w365 {
            tunnel: w377 -> [_ w387]
            tunnel: w375 -> [w379 w386]
            tunnel: [w379 w385] -> w374
            tunnel: w373 -> [_ w384]
            tunnel: w371 -> [_ w383]
            tunnel: w370 -> [_ w382]
            tunnel: [_ w381] -> w369
            tunnel: w368 -> [_ w380]
            frame False {
            }
            frame True {
              n211 = case shown="1..8" w380 {
                tunnel: w387 -> [_ w392 w407]
                tunnel: w386 -> [w388 w390 w404]
                tunnel: [w388 w391 w403] -> w385
                tunnel: w383 -> [_ w393 w406]
                tunnel: w384 -> [_ w396 _]
                tunnel: w382 -> [_ w395 w405]
                tunnel: [_ _ w402] -> w381
                frame Default {
                  # "INCOMPATIBLE DATATYPES"
                }
                frame 112 {
                  # "Check if subtype matches"
                  # "REFNUM - CHECK SUBTYPE"
                  n212 = Index Array(array=w396, index=2) -> (element=w394:i16)
                  n213 = Equal?(x=w395, y=w394) -> (x = y?=w389:bool)
                  n214 = case shown="True" w389 {
                    tunnel: w393 -> [_ w401]
                    tunnel: w392 -> [_ w400]
                    tunnel: [w398 w399] -> w391
                    tunnel: w390 -> [w398 _]
                    frame False {
                    }
                    frame True {
                      n215 = Flattened String To Variant(6:w400, 7:w401) -> (3:w399:variant)  [unwired: 1 in, 1 out]
                    }
                  }
                }
                frame 1..8 {
                  # "4-byte types or higher resolution"
                  n216 = case shown="1, 4, 8, 9, 11, 12, 14, 15, 17, 19" w405 {
                    tunnel: w407 -> [_ w418]
                    tunnel: w406 -> [_ w412]
                    tunnel: w404 -> [w408 _]
                    tunnel: [w408 w410] -> w403
                    tunnel: [_ TRUE] -> w402
                    frame Default {
                    }
                    frame 1, 4, 8, 9, 17, 18, 20, 21, 23, 25 {
                      # "Any types that have at least\n4 bytes."
                      n217 = String To Byte Array(string=w418) -> (unsigned byte array=w417:u8[])
                      n218 = Reverse 1D Array(array=w417) -> (reversed array=w416:u8[])
                      n219 = Array Subset(array=w416, length=4) -> (w414:u8[])  [unwired: 1 in]
                      n220 = Reverse 1D Array(array=w414) -> (reversed array=w413:u8[])
                      n221 = Byte Array To String(unsigned byte array=w413) -> (string=w411:string)
                      n222 = Flattened String To Variant(6:w411, 7:w412) -> (3:w410:variant)  [unwired: 1 in, 1 out]
                    }
                  }
                }
              }
            }
          }
        }
      }
    }
    frame Enabled {
    }
  }
